vi "ClassError.vi"(7 "Kill":bool, 8 "error in (no error)":errorcluster, 9 "Text":string, 10 "From":string, 11 "error in":errorcluster) -> (0 "error out":errorcluster)   [LabVIEW 2017, in "Error.lvlib"]
doc: "Write data to main coms q for module (generic)"
uses:
  Error.lvlib
  ctl/MainData.ctl
  ctl/MainStates.ctl
  ctl/ErrorInfo.ctl
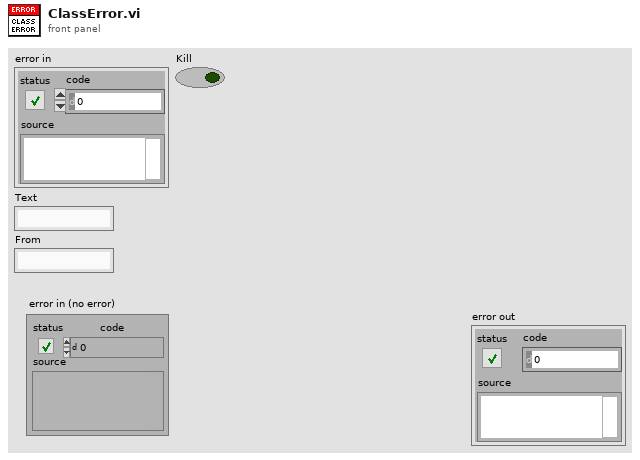
[diagram p1: front panel]
types:
  T1 = typedef "Error.lvlib/ErrorInfo.ctl" = cluster{"error in":errorcluster, "Text":string, "From":string, "Kill":bool}
  T2 = typedef "Error.lvlib/MainStates.ctl" = enum16{"Timeout", "Error", "Exit", "Init", "ClassError", "LogError", "Shutdown", "Warning"}
  T3 = typedef "Error.lvlib/MainData.ctl" = cluster{"State":T2, "Variant":variant}
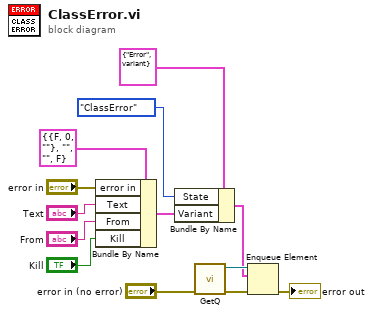
[diagram p0: block diagram]
diagram:
  n1 = Bundle By Name(cluster=T1 {"error in"={"status"=FALSE, "code"=0, "source"=""}, "Text"="", "From"="", "Kill"=FALSE} ("Error info"), "error in"="error in", "Text"="Text", "From"="From", "Kill"="Kill") -> (w5:T1)
  n2 = Bundle By Name(cluster=T3 {"State"=enum."Error", "Variant"=variant} ("Data"), "State"=MainStates."ClassError", "Variant"=w5) -> (w9:T3)
  n3 = call "GetQ.vi"("error in (no error)"="error in (no error)") -> ("error out"=w12:errorcluster, "Q out"=w13:refnum<queue>)  [unwired: 9 in]
  n4 = Enqueue Element(queue=w13, element=w9, error in (no error)=w12) -> (error out=→"error out":errorcluster)  [unwired: 1 in, 2 out]
